vi "Prepare Glue.vi"(7 "Console Log in":refnum<class "Console Log.lvclass">, 8 "error in":errorcluster, 11 "Gluing Procedure in":refnum<class "Gluing Procedure.lvclass">) -> (0 "error out":errorcluster, 1 "Step canceled?":bool, 3 "Gluing Procedure out":refnum<class "Gluing Procedure.lvclass">, 5 "Console Log out":refnum<class "Console Log.lvclass">)   [LabVIEW 2011]
uses:
  Procedure Classes/Gluing Procedure/Gluing Procedure.lvclass
  Application Utilities/Console Log/Console Log.lvclass
  Shared Components/WorkTable Class/WorkTable Class.lvclass
  Procedure Classes/Gluing Procedure/Type Definitions/Prepare Glue.ctl
panel:
  out "Glue Slots":string[](array[string])
  in  "Cancel Button":bool
  in  "OK Button":bool
  in  "Glue Prep Time":timestamp=timestamp(3550680760.677781 s since 1904-01-01)
  # "Prepare glue!\n\nPlace on glue resevoir slot(s) being used.\n\nEnter the approximate time of glue preperation here, or use the current time."
  # "This VI simply prompts the user to prepare the glue before operation of the main gluing motion"
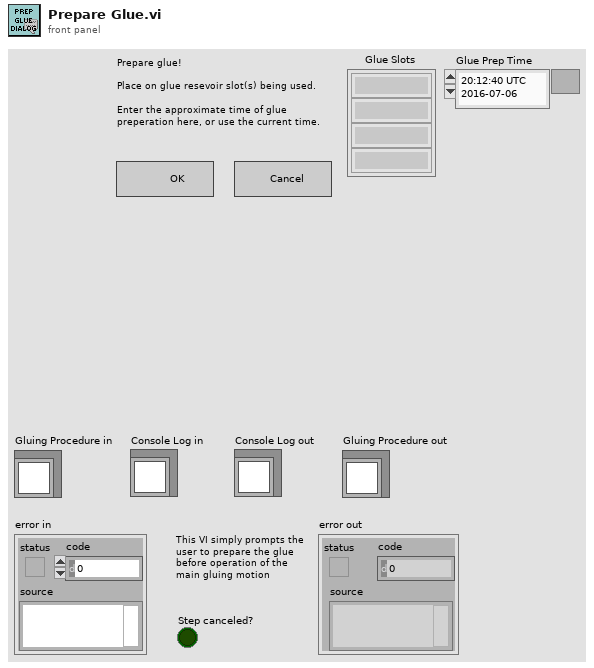
[diagram p1: front panel]
types:
  T1 = typedef "Worktable_Glue Reservoir.ctl" = cluster{"Glue Reservoir Slots":cluster{"Reservoir State":enum16{"Empty", "Full", "Used"}, "Center":refnum<class "Vec3d Class.lvclass">}[], "Vacuum Channel":i32}
  T2 = cluster{"Reservoir State":enum16{"Empty", "Full", "Used"}, "Center":refnum<class "Vec3d Class.lvclass">}[]
  T3 = typedef "Prepare Glue.ctl" = cluster{"Has been run?":bool}
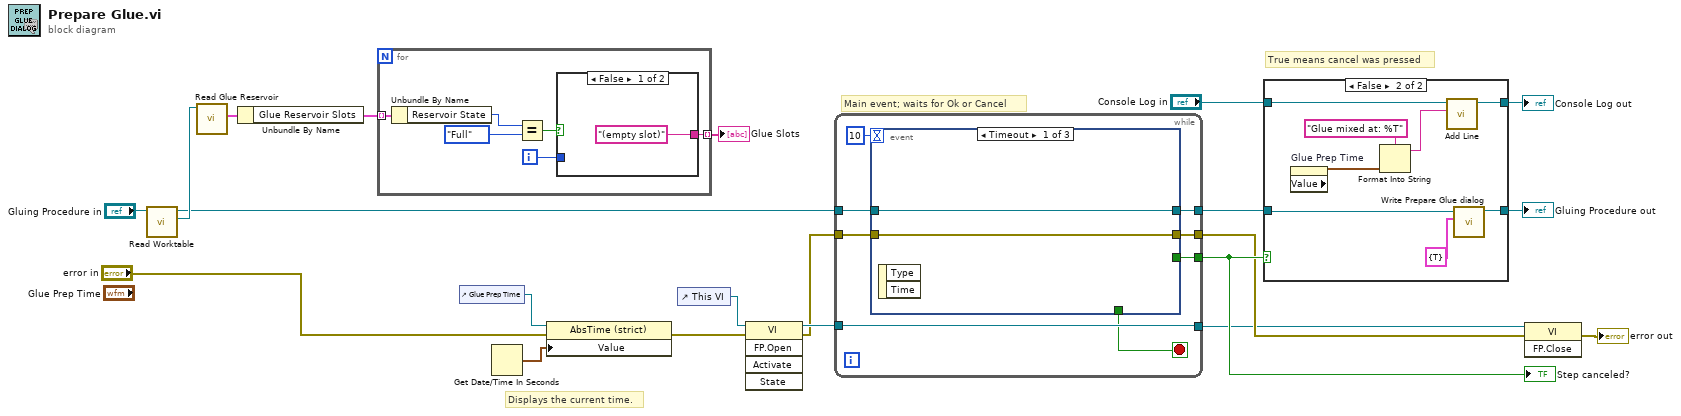
[diagram p0: block diagram]
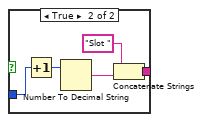
[diagram p2: hidden frame]
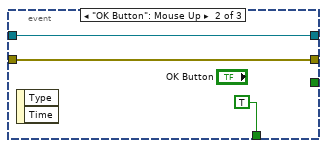
[diagram p4: hidden frame]
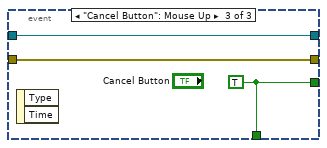
[diagram p5: hidden frame]
diagram:
  # "Displays the current time."
  # "Main event; waits for Ok or Cancel"
  # "True means cancel was pressed"
  n1 = call "Read Worktable.vi"("Gluing Procedure in"="Gluing Procedure in") -> ("WorkTable out"=w6:refnum<class "WorkTable Class.lvclass">, "Gluing Procedure out"=w1:refnum<class "Gluing Procedure.lvclass">)  [unwired: 8 in, 1 out]
  n2 = call-dynamic "Read Glue Reservoir.vi"("WorkTable Class in"=w6) -> ("Glue Reservoir"=w5:T1)  [unwired: 8 in, 2 out]
  n3 = Unbundle By Name(w5) -> ("Glue Reservoir Slots"=w4:T2)
  n4 = for {
    tunnel: w4 -> [w27] mode=indexing
    tunnel: [w22] -> w3 mode=indexing
    i -> [w23]
    n5 = Unbundle By Name(w27) -> ("Reservoir State"=w26:enum16{"Empty", "Full", "Used"})
    n6 = Equal?(x=w26, y=enum16{"Empty", "Full", "Used"}."Full") -> (x = y?=w24:bool)
    n7 = case shown="False" w24 {
      tunnel: w23 -> [_ w30]
      tunnel: ["(empty slot)" w29] -> w22
      frame False {
      }
      frame True {
        n8 = Increment(x=w30) -> (x+1=w31:i32)
        n9 = Number To Decimal String(number=w31) -> (decimal integer string=w33:string)  [unwired: 1 in]
        n10 = Concatenate Strings("Slot " ("format string"), w33) -> (w29:string)
      }
    }
  }
  "Glue Slots" <- w3
  n11 = control-ref of="Glue Prep Time"() -> (w16:refnum<vi>)
  n12 = Get Date/Time In Seconds() -> (seconds since 1Jan1904=w15:timestamp)
  n13 = property class="AbsTime (strict)"(reference=w16, error in="error in", "Value"=w15) -> (error out=w13:errorcluster)  [unwired: 1 out]
  n14 = control-ref of="This VI"() -> (w21:refnum<vi>)
  n15 = invoke class="VI" method="FP.Open"(reference=w21, error in=w13) -> (reference out=w20:refnum<vi>, error out=w12:errorcluster)  [unwired: 3 in, 3 out]
  n16 = while {
    tunnel: w1 -> [w40]
    tunnel: [w39] -> w18
    tunnel: w12 -> [w38]
    tunnel: [w37] -> w9
    tunnel: w20 -> [w41]
    tunnel: [w41] -> w7
    tunnel: [w34] -> w11
    stop <- w35 stop-if-true
    n17 = event shown="[0] Timeout" {
      selector: _ -> [_ _ _]
      dyn-events: _ -> [_ _ _]
      timeout: 10 -> [_ _ _]
      tunnel: w40 -> [w43 w45 w49]
      tunnel: [w43 w45 w49] -> w39
      tunnel: w38 -> [w42 w44 w48]
      tunnel: [w42 w44 w48] -> w37
      tunnel: [_ TRUE w47] -> w35
      tunnel: [_ _ w47] -> w34
      event Timeout {
        n18 = event-data() -> ()  [unwired: 1 in, 2 out]
      }
      event "OK Button": Mouse Up {
        n19 = event-data() -> ()  [unwired: 1 in, 2 out]
      }
      event "Cancel Button": Mouse Up {
        w47 = TRUE
        n20 = event-data() -> ()  [unwired: 1 in, 2 out]
      }
    }
  }
  "Step canceled?" <- w11
  n21 = case shown="False" w11 {
    tunnel: [w50 w59] -> w19
    tunnel: w18 -> [w50 w52]
    tunnel: "Console Log in" -> [w51 w53]
    tunnel: [w51 w57] -> w17
    frame True {
    }
    frame False {
      n22 = property on="Glue Prep Time" class="AbsTime (strict)"() -> ("Value"=w55:timestamp)  [unwired: 2 in, 2 out]
      n23 = Format Into String(format string="Glue mixed at: %T", w55) -> (resulting string=w56:string)  [unwired: 2 in, 1 out]
      n24 = call "Add Line.vi"("String"=w56, "Console Log in"=w53) -> ("Console Log out"=w57:refnum<class "Console Log.lvclass">)  [unwired: 8 in, 1 out]
      n25 = call "Write Prepare Glue dialog.vi"("Prepare Glue dialog"=T3 {"Has been run?"=TRUE}, "Gluing Procedure in"=w52) -> ("Gluing Procedure out"=w59:refnum<class "Gluing Procedure.lvclass">)  [unwired: 8 in, 1 out]
    }
  }
  "Gluing Procedure out" <- w19
  "Console Log out" <- w17
  n26 = invoke class="VI" method="FP.Close"(reference=w7, error in=w9) -> (error out=→"error out":errorcluster)  [unwired: 1 in, 2 out]
